vi "LAMMPS Animation.vi"() -> ()   [LabVIEW 2010]
uses:
  <vilib>/picture/3D Picture Control/NI_3D Picture Control.lvlib
panel:
  out "element":T1
  in  "Path":path
  in  "Options":cluster{"Border?":bool, "Bonds?":bool}
  out "Scene Display":refnum<vi>(3d-picture)
  in  "Scale":dbl(slide)=0.03473491773308958 scale=0.0..0.2
  in  "Atom Size":dbl=0.75
  out "Base Object":refnum<vi>
  in  "Slide":i32(slide) scale=0.0..22.0
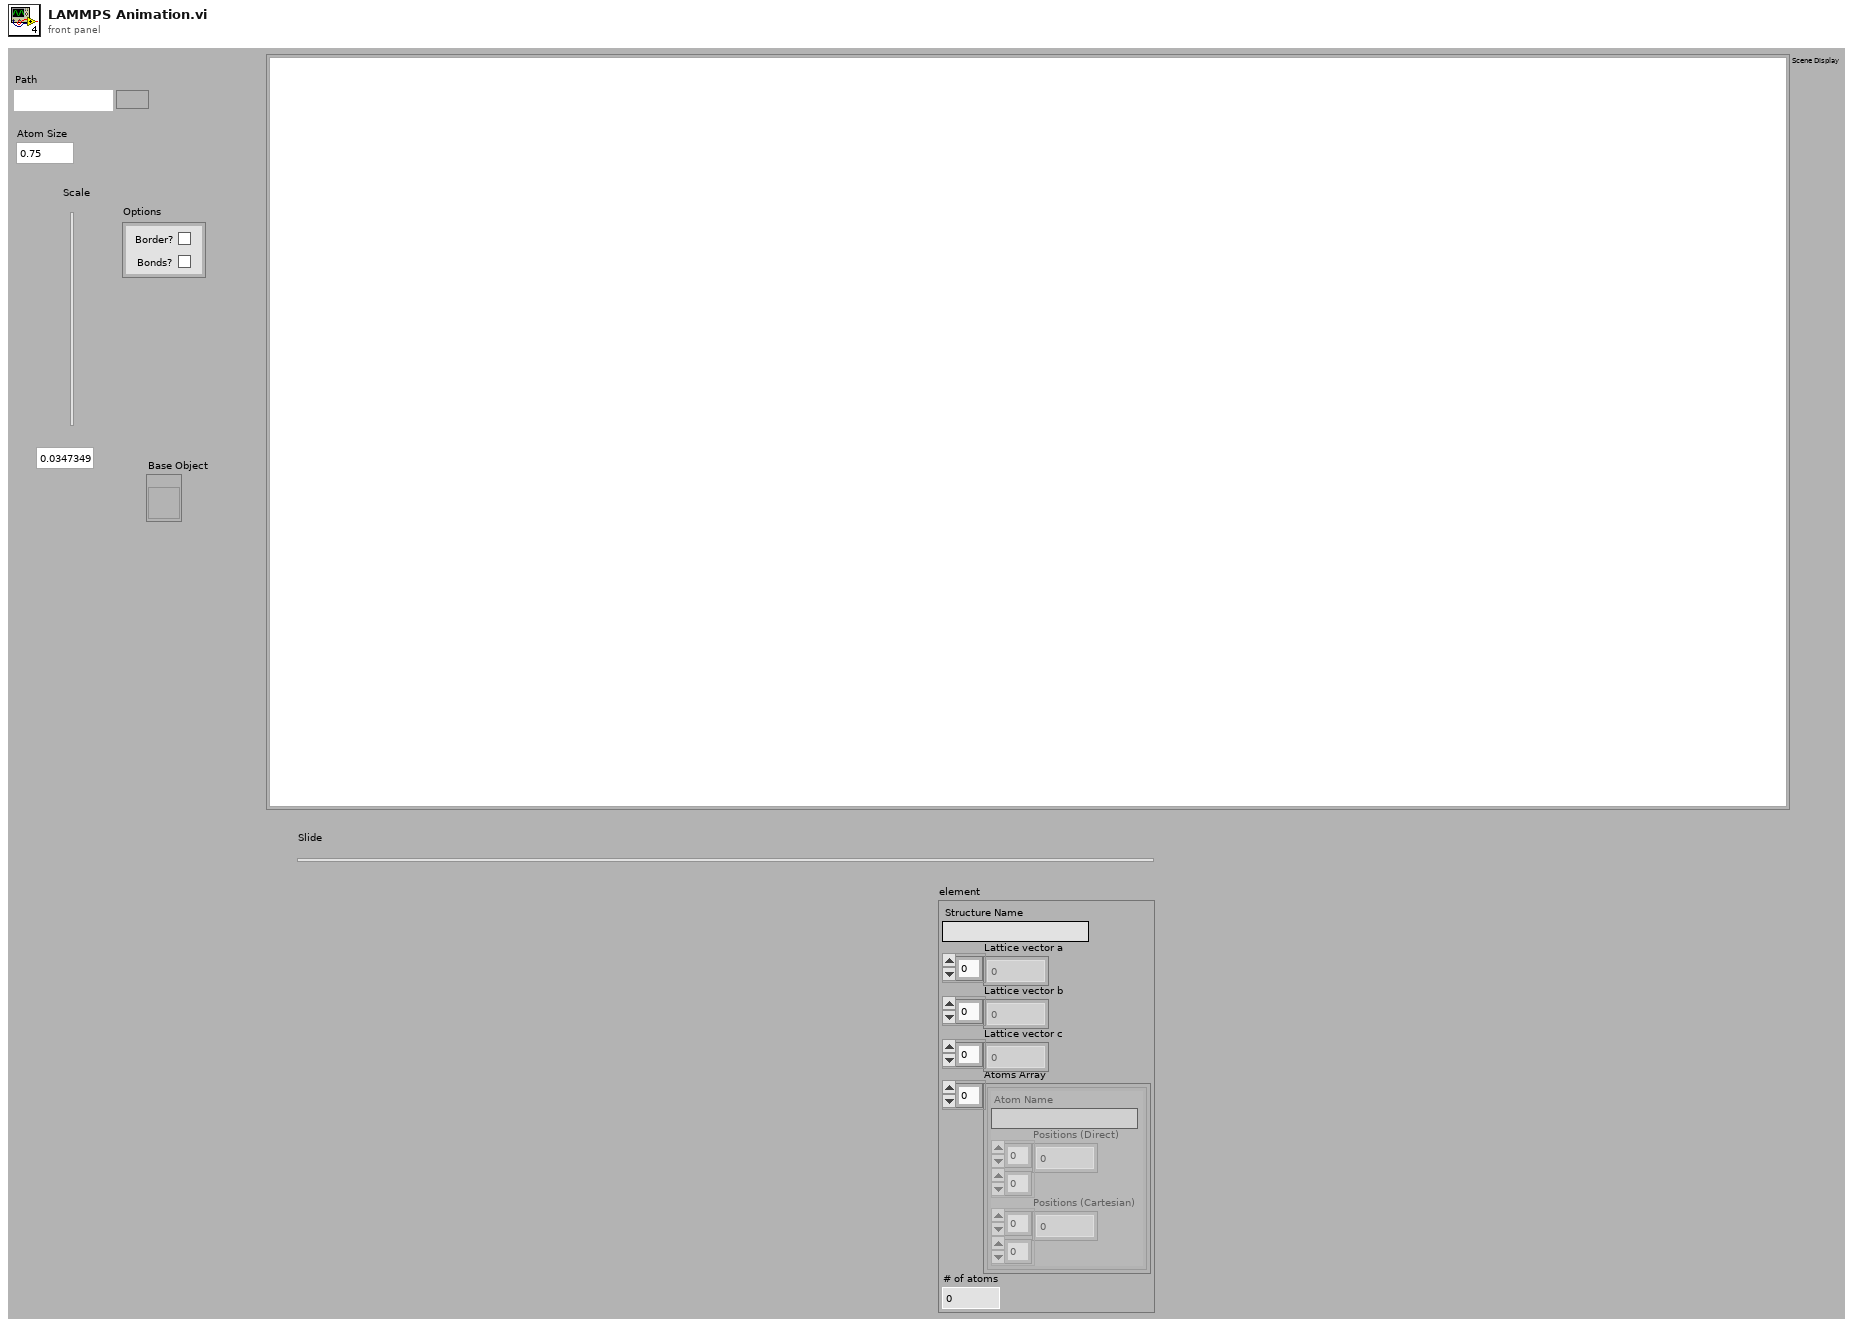
[diagram p1: front panel]
types:
  T1 = cluster{"Structure Name":string, "Lattice vector a":dbl[], "Lattice vector b":dbl[], "Lattice vector c":dbl[], "Atoms Array":cluster{"Atom Name":string, "Positions (Direct)":dbl[][], "Positions (Cartesian)":dbl[][]}[], "# of atoms":i32}
  T2 = cluster{"Structure Name":string, "Lattice vector a":dbl[], "Lattice vector b":dbl[], "Lattice vector c":dbl[], "Atoms Array":cluster{"Atom Name":string, "Positions (Direct)":dbl[][], "Positions (Cartesian)":dbl[][]}[], "# of atoms":i32}[]
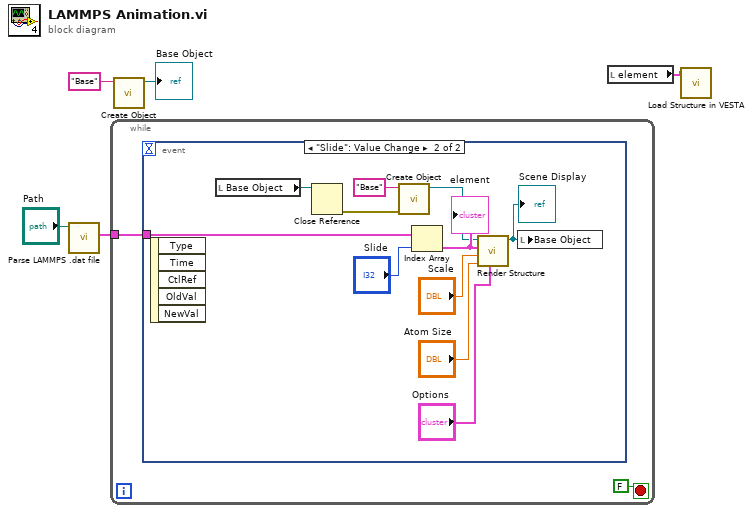
[diagram p0: block diagram]
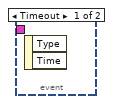
[diagram p2: hidden frame]
diagram:
  n1 = call "Parse LAMMPS .dat file.vi"("Path"="Path") -> ("Structures Array"=w5:T2)  [unwired: 9 in, 1 out]
  n2 = while {
    tunnel: w5 -> [w6]
    stop <- FALSE stop-if-true
    n3 = event shown="[1] \"Slide\": Value Change" {
      selector: _ -> [_ _]
      dyn-events: _ -> [_ _]
      timeout: _ -> [_ _]
      tunnel: w6 -> [_ w17]
      event Timeout {
        n4 = event-data() -> ()  [unwired: 1 in, 2 out]
      }
      event "Slide": Value Change {
        n5 = event-data() -> ()  [unwired: 1 in, 5 out]
        n6 = local read "Base Object"() -> (w8:refnum<vi>)
        n7 = Close Reference(reference=w8) -> (error out=w11:errorcluster)  [unwired: 1 in]
        n8 = call <vilib>:"Create Object.vi"("error in (no error)"=w11, "Name"="Base") -> ("Scene:New Object"=w9:refnum<vi>)  [unwired: 9 out]
        n9 = Index Array(array=w17, index="Slide") -> (element=w16:T1)
        "element" <- w16
        n10 = call "Render Structure.vi"("Options"="Options", "Atom Size"="Atom Size", "Scale"="Scale", "Atomic Structure"=w16, "Base Object"=w9) -> ("Object with atoms"=w13:refnum<vi>)  [unwired: 6 in]
        "Scene Display" <- w13
        n11 = local write "Base Object"(w13) -> ()
      }
    }
  }
  n12 = call <vilib>:"Create Object.vi"("Name"="Base") -> ("Scene:New Object"=→"Base Object":refnum<vi>)  [unwired: 1 in, 9 out]
  n13 = local read "element"() -> (w1:T1)
  n14 = call "Load Structure in VESTA.vi"("Atomic Structure"=w1) -> ()  [unwired: 11 in]
